vi "PCO_Camera_Type.vi"() -> (0 "PCO_CameraType":T1 {"wCamType" format="%x"; "wCamSubType" format="%x"; "InterfaceType" format="%x"}, 1 "PCO_CameraType_Raw":T2, 2 "Length":u16, 3 "Raw_Length":u16)   [LabVIEW 2019, in "SDK.lvlib" / "Structures.lvlib"]
doc: "Use this template to build a VI to use as a subVI."
uses:
  Structures.lvlib
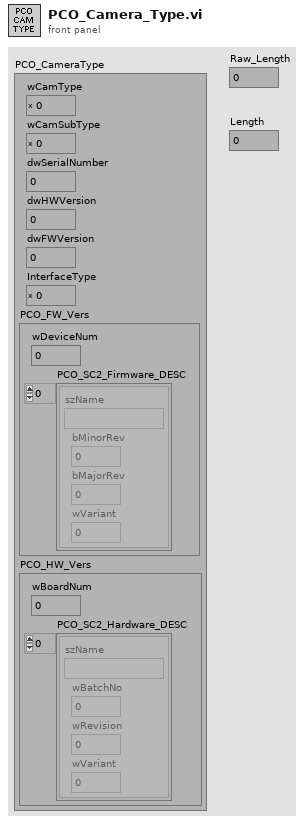
[diagram p1: front panel]
types:
  T1 = cluster{"wCamType":u16, "wCamSubType":u16, "dwSerialNumber":u32, "dwHWVersion":u32, "dwFWVersion":u32, "InterfaceType":u16, "PCO_FW_Vers":cluster{"wDeviceNum":u16, "PCO_SC2_Firmware_DESC":cluster{"szName":string, "bMinorRev":u8, "bMajorRev":u8, "wVariant":u16}[]}, "PCO_HW_Vers":cluster{"wBoardNum":u16, "PCO_SC2_Hardware_DESC":cluster{"szName":string, "wBatchNo":u16, "wRevision":u16, "wVariant":u16}[]}}
  T2 = cluster{"wSize":u16, "wCamType":u16, "wCamSubType":u16, "zzwAlignDummy1":u16, "dwSerialNumber":u32, "dwHWVersion":u32, "dwFWVersion":u32, "wInterfaceType":u16, "PCO_FW_Vers_Raw":cluster{"wDeviceNum":u16, "PCO_SC2_Firmware_DESC":cluster{"PCO_SC2_FW_Desc_Raw":cluster{"szName":cluster{u8, u8, u8, u8, u8, u8, u8, u8, u8, u8, u8, u8, u8, u8, u8, u8}, "bMinorRev":u8, "bMajorRev":u8, "wVariant":u16, "zzwDummy":cluster{u16, u16, u16, u16, u16, u16, u16, u16, u16, u16, u16, u16, u16, u16, u16, u16, u16, u16, u16, u16, u16, u16}}, "PCO_SC2_FW_Desc_Raw":cluster{"szName":cluster{u8, u8, u8, u8, u8, u8, u8, u8, u8, u8, u8, u8, u8, u8, u8, u8}, "bMinorRev":u8, "bMajorRev":u8, "wVariant":u16, "zzwDummy":cluster{u16, u16, u16, u16, u16, u16, u16, u16, u16, u16, u16, u16, u16, u16, u16, u16, u16, u16, u16, u16, u16, u16}}, "PCO_SC2_FW_Desc_Raw":cluster{"szName":cluster{u8, u8, u8, u8, u8, u8, u8, u8, u8, u8, u8, u8, u8, u8, u8, u8}, "bMinorRev":u8, "bMajorRev":u8, "wVariant":u16, "zzwDummy":cluster{u16, u16, u16, u16, u16, u16, u16, u16, u16, u16, u16, u16, u16, u16, u16, u16, u16, u16, u16, u16, u16, u16}}, "PCO_SC2_FW_Desc_Raw":cluster{"szName":cluster{u8, u8, u8, u8, u8, u8, u8, u8, u8, u8, u8, u8, u8, u8, u8, u8}, "bMinorRev":u8, "bMajorRev":u8, "wVariant":u16, "zzwDummy":cluster{u16, u16, u16, u16, u16, u16, u16, u16, u16, u16, u16, u16, u16, u16, u16, u16, u16, u16, u16, u16, u16, u16}}, "PCO_SC2_FW_Desc_Raw":cluster{"szName":cluster{u8, u8, u8, u8, u8, u8, u8, u8, u8, u8, u8, u8, u8, u8, u8, u8}, "bMinorRev":u8, "bMajorRev":u8, "wVariant":u16, "zzwDummy":cluster{u16, u16, u16, u16, u16, u16, u16, u16, u16, u16, u16, u16, u16, u16, u16, u16, u16, u16, u16, u16, u16, u16}}, "PCO_SC2_FW_Desc_Raw":cluster{"szName":cluster{u8, u8, u8, u8, u8, u8, u8, u8, u8, u8, u8, u8, u8, u8, u8, u8}, "bMinorRev":u8, "bMajorRev":u8, "wVariant":u16, "zzwDummy":cluster{u16, u16, u16, u16, u16, u16, u16, u16, u16, u16, u16, u16, u16, u16, u16, u16, u16, u16, u16, u16, u16, u16}}, "PCO_SC2_FW_Desc_Raw":cluster{"szName":cluster{u8, u8, u8, u8, u8, u8, u8, u8, u8, u8, u8, u8, u8, u8, u8, u8}, "bMinorRev":u8, "bMajorRev":u8, "wVariant":u16, "zzwDummy":cluster{u16, u16, u16, u16, u16, u16, u16, u16, u16, u16, u16, u16, u16, u16, u16, u16, u16, u16, u16, u16, u16, u16}}, "PCO_SC2_FW_Desc_Raw":cluster{"szName":cluster{u8, u8, u8, u8, u8, u8, u8, u8, u8, u8, u8, u8, u8, u8, u8, u8}, "bMinorRev":u8, "bMajorRev":u8, "wVariant":u16, "zzwDummy":cluster{u16, u16, u16, u16, u16, u16, u16, u16, u16, u16, u16, u16, u16, u16, u16, u16, u16, u16, u16, u16, u16, u16}}, "PCO_SC2_FW_Desc_Raw":cluster{"szName":cluster{u8, u8, u8, u8, u8, u8, u8, u8, u8, u8, u8, u8, u8, u8, u8, u8}, "bMinorRev":u8, "bMajorRev":u8, "wVariant":u16, "zzwDummy":cluster{u16, u16, u16, u16, u16, u16, u16, u16, u16, u16, u16, u16, u16, u16, u16, u16, u16, u16, u16, u16, u16, u16}}, "PCO_SC2_FW_Desc_Raw":cluster{"szName":cluster{u8, u8, u8, u8, u8, u8, u8, u8, u8, u8, u8, u8, u8, u8, u8, u8}, "bMinorRev":u8, "bMajorRev":u8, "wVariant":u16, "zzwDummy":cluster{u16, u16, u16, u16, u16, u16, u16, u16, u16, u16, u16, u16, u16, u16, u16, u16, u16, u16, u16, u16, u16, u16}}}}, "PCO_HW_Vers_Raw":cluster{"wBoardNum":u16, "PCO_SC2_Hardware_DESC":cluster{"PCO_SC2_HW_Desc_Raw":cluster{"szName":cluster{u8, u8, u8, u8, u8, u8, u8, u8, u8, u8, u8, u8, u8, u8, u8, u8}, "wBatchNo":u16, "wRevision":u16, "wVariant":u16, "zzwDummy":cluster{u16, u16, u16, u16, u16, u16, u16, u16, u16, u16, u16, u16, u16, u16, u16, u16, u16, u16, u16, u16}}, "PCO_SC2_HW_Desc_Raw":cluster{"szName":cluster{u8, u8, u8, u8, u8, u8, u8, u8, u8, u8, u8, u8, u8, u8, u8, u8}, "wBatchNo":u16, "wRevision":u16, "wVariant":u16, "zzwDummy":cluster{u16, u16, u16, u16, u16, u16, u16, u16, u16, u16, u16, u16, u16, u16, u16, u16, u16, u16, u16, u16}}, "PCO_SC2_HW_Desc_Raw":cluster{"szName":cluster{u8, u8, u8, u8, u8, u8, u8, u8, u8, u8, u8, u8, u8, u8, u8, u8}, "wBatchNo":u16, "wRevision":u16, "wVariant":u16, "zzwDummy":cluster{u16, u16, u16, u16, u16, u16, u16, u16, u16, u16, u16, u16, u16, u16, u16, u16, u16, u16, u16, u16}}, "PCO_SC2_HW_Desc_Raw":cluster{"szName":cluster{u8, u8, u8, u8, u8, u8, u8, u8, u8, u8, u8, u8, u8, u8, u8, u8}, "wBatchNo":u16, "wRevision":u16, "wVariant":u16, "zzwDummy":cluster{u16, u16, u16, u16, u16, u16, u16, u16, u16, u16, u16, u16, u16, u16, u16, u16, u16, u16, u16, u16}}, "PCO_SC2_HW_Desc_Raw":cluster{"szName":cluster{u8, u8, u8, u8, u8, u8, u8, u8, u8, u8, u8, u8, u8, u8, u8, u8}, "wBatchNo":u16, "wRevision":u16, "wVariant":u16, "zzwDummy":cluster{u16, u16, u16, u16, u16, u16, u16, u16, u16, u16, u16, u16, u16, u16, u16, u16, u16, u16, u16, u16}}, "PCO_SC2_HW_Desc_Raw":cluster{"szName":cluster{u8, u8, u8, u8, u8, u8, u8, u8, u8, u8, u8, u8, u8, u8, u8, u8}, "wBatchNo":u16, "wRevision":u16, "wVariant":u16, "zzwDummy":cluster{u16, u16, u16, u16, u16, u16, u16, u16, u16, u16, u16, u16, u16, u16, u16, u16, u16, u16, u16, u16}}, "PCO_SC2_HW_Desc_Raw":cluster{"szName":cluster{u8, u8, u8, u8, u8, u8, u8, u8, u8, u8, u8, u8, u8, u8, u8, u8}, "wBatchNo":u16, "wRevision":u16, "wVariant":u16, "zzwDummy":cluster{u16, u16, u16, u16, u16, u16, u16, u16, u16, u16, u16, u16, u16, u16, u16, u16, u16, u16, u16, u16}}, "PCO_SC2_HW_Desc_Raw":cluster{"szName":cluster{u8, u8, u8, u8, u8, u8, u8, u8, u8, u8, u8, u8, u8, u8, u8, u8}, "wBatchNo":u16, "wRevision":u16, "wVariant":u16, "zzwDummy":cluster{u16, u16, u16, u16, u16, u16, u16, u16, u16, u16, u16, u16, u16, u16, u16, u16, u16, u16, u16, u16}}, "PCO_SC2_HW_Desc_Raw":cluster{"szName":cluster{u8, u8, u8, u8, u8, u8, u8, u8, u8, u8, u8, u8, u8, u8, u8, u8}, "wBatchNo":u16, "wRevision":u16, "wVariant":u16, "zzwDummy":cluster{u16, u16, u16, u16, u16, u16, u16, u16, u16, u16, u16, u16, u16, u16, u16, u16, u16, u16, u16, u16}}, "PCO_SC2_HW_Desc_Raw":cluster{"szName":cluster{u8, u8, u8, u8, u8, u8, u8, u8, u8, u8, u8, u8, u8, u8, u8, u8}, "wBatchNo":u16, "wRevision":u16, "wVariant":u16, "zzwDummy":cluster{u16, u16, u16, u16, u16, u16, u16, u16, u16, u16, u16, u16, u16, u16, u16, u16, u16, u16, u16, u16}}}}, "zzWDummy":cluster{u16, u16, u16, u16, u16, u16, u16, u16, u16, u16, u16, u16, u16, u16, u16, u16, u16, u16, u16, u16, u16, u16, u16, u16, u16, u16, u16, u16, u16, u16, u16, u16, u16, u16, u16, u16, u16, u16, u16}}
  T3 = cluster{u16, u16, u16, u16, u16, u16, u16, u16, u16, u16, u16, u16, u16, u16, u16, u16, u16, u16, u16, u16, u16, u16, u16, u16, u16, u16, u16, u16, u16, u16, u16, u16, u16, u16, u16, u16, u16, u16, u16}
  T4 = cluster{"wDeviceNum":u16, "PCO_SC2_Firmware_DESC":cluster{"szName":string, "bMinorRev":u8, "bMajorRev":u8, "wVariant":u16}[]}
  T5 = cluster{"wDeviceNum":u16, "PCO_SC2_Firmware_DESC":cluster{"PCO_SC2_FW_Desc_Raw":cluster{"szName":cluster{u8, u8, u8, u8, u8, u8, u8, u8, u8, u8, u8, u8, u8, u8, u8, u8}, "bMinorRev":u8, "bMajorRev":u8, "wVariant":u16, "zzwDummy":cluster{u16, u16, u16, u16, u16, u16, u16, u16, u16, u16, u16, u16, u16, u16, u16, u16, u16, u16, u16, u16, u16, u16}}, "PCO_SC2_FW_Desc_Raw":cluster{"szName":cluster{u8, u8, u8, u8, u8, u8, u8, u8, u8, u8, u8, u8, u8, u8, u8, u8}, "bMinorRev":u8, "bMajorRev":u8, "wVariant":u16, "zzwDummy":cluster{u16, u16, u16, u16, u16, u16, u16, u16, u16, u16, u16, u16, u16, u16, u16, u16, u16, u16, u16, u16, u16, u16}}, "PCO_SC2_FW_Desc_Raw":cluster{"szName":cluster{u8, u8, u8, u8, u8, u8, u8, u8, u8, u8, u8, u8, u8, u8, u8, u8}, "bMinorRev":u8, "bMajorRev":u8, "wVariant":u16, "zzwDummy":cluster{u16, u16, u16, u16, u16, u16, u16, u16, u16, u16, u16, u16, u16, u16, u16, u16, u16, u16, u16, u16, u16, u16}}, "PCO_SC2_FW_Desc_Raw":cluster{"szName":cluster{u8, u8, u8, u8, u8, u8, u8, u8, u8, u8, u8, u8, u8, u8, u8, u8}, "bMinorRev":u8, "bMajorRev":u8, "wVariant":u16, "zzwDummy":cluster{u16, u16, u16, u16, u16, u16, u16, u16, u16, u16, u16, u16, u16, u16, u16, u16, u16, u16, u16, u16, u16, u16}}, "PCO_SC2_FW_Desc_Raw":cluster{"szName":cluster{u8, u8, u8, u8, u8, u8, u8, u8, u8, u8, u8, u8, u8, u8, u8, u8}, "bMinorRev":u8, "bMajorRev":u8, "wVariant":u16, "zzwDummy":cluster{u16, u16, u16, u16, u16, u16, u16, u16, u16, u16, u16, u16, u16, u16, u16, u16, u16, u16, u16, u16, u16, u16}}, "PCO_SC2_FW_Desc_Raw":cluster{"szName":cluster{u8, u8, u8, u8, u8, u8, u8, u8, u8, u8, u8, u8, u8, u8, u8, u8}, "bMinorRev":u8, "bMajorRev":u8, "wVariant":u16, "zzwDummy":cluster{u16, u16, u16, u16, u16, u16, u16, u16, u16, u16, u16, u16, u16, u16, u16, u16, u16, u16, u16, u16, u16, u16}}, "PCO_SC2_FW_Desc_Raw":cluster{"szName":cluster{u8, u8, u8, u8, u8, u8, u8, u8, u8, u8, u8, u8, u8, u8, u8, u8}, "bMinorRev":u8, "bMajorRev":u8, "wVariant":u16, "zzwDummy":cluster{u16, u16, u16, u16, u16, u16, u16, u16, u16, u16, u16, u16, u16, u16, u16, u16, u16, u16, u16, u16, u16, u16}}, "PCO_SC2_FW_Desc_Raw":cluster{"szName":cluster{u8, u8, u8, u8, u8, u8, u8, u8, u8, u8, u8, u8, u8, u8, u8, u8}, "bMinorRev":u8, "bMajorRev":u8, "wVariant":u16, "zzwDummy":cluster{u16, u16, u16, u16, u16, u16, u16, u16, u16, u16, u16, u16, u16, u16, u16, u16, u16, u16, u16, u16, u16, u16}}, "PCO_SC2_FW_Desc_Raw":cluster{"szName":cluster{u8, u8, u8, u8, u8, u8, u8, u8, u8, u8, u8, u8, u8, u8, u8, u8}, "bMinorRev":u8, "bMajorRev":u8, "wVariant":u16, "zzwDummy":cluster{u16, u16, u16, u16, u16, u16, u16, u16, u16, u16, u16, u16, u16, u16, u16, u16, u16, u16, u16, u16, u16, u16}}, "PCO_SC2_FW_Desc_Raw":cluster{"szName":cluster{u8, u8, u8, u8, u8, u8, u8, u8, u8, u8, u8, u8, u8, u8, u8, u8}, "bMinorRev":u8, "bMajorRev":u8, "wVariant":u16, "zzwDummy":cluster{u16, u16, u16, u16, u16, u16, u16, u16, u16, u16, u16, u16, u16, u16, u16, u16, u16, u16, u16, u16, u16, u16}}}}
  T6 = cluster{"wBoardNum":u16, "PCO_SC2_Hardware_DESC":cluster{"szName":string, "wBatchNo":u16, "wRevision":u16, "wVariant":u16}[]}
  T7 = cluster{"wBoardNum":u16, "PCO_SC2_Hardware_DESC":cluster{"PCO_SC2_HW_Desc_Raw":cluster{"szName":cluster{u8, u8, u8, u8, u8, u8, u8, u8, u8, u8, u8, u8, u8, u8, u8, u8}, "wBatchNo":u16, "wRevision":u16, "wVariant":u16, "zzwDummy":cluster{u16, u16, u16, u16, u16, u16, u16, u16, u16, u16, u16, u16, u16, u16, u16, u16, u16, u16, u16, u16}}, "PCO_SC2_HW_Desc_Raw":cluster{"szName":cluster{u8, u8, u8, u8, u8, u8, u8, u8, u8, u8, u8, u8, u8, u8, u8, u8}, "wBatchNo":u16, "wRevision":u16, "wVariant":u16, "zzwDummy":cluster{u16, u16, u16, u16, u16, u16, u16, u16, u16, u16, u16, u16, u16, u16, u16, u16, u16, u16, u16, u16}}, "PCO_SC2_HW_Desc_Raw":cluster{"szName":cluster{u8, u8, u8, u8, u8, u8, u8, u8, u8, u8, u8, u8, u8, u8, u8, u8}, "wBatchNo":u16, "wRevision":u16, "wVariant":u16, "zzwDummy":cluster{u16, u16, u16, u16, u16, u16, u16, u16, u16, u16, u16, u16, u16, u16, u16, u16, u16, u16, u16, u16}}, "PCO_SC2_HW_Desc_Raw":cluster{"szName":cluster{u8, u8, u8, u8, u8, u8, u8, u8, u8, u8, u8, u8, u8, u8, u8, u8}, "wBatchNo":u16, "wRevision":u16, "wVariant":u16, "zzwDummy":cluster{u16, u16, u16, u16, u16, u16, u16, u16, u16, u16, u16, u16, u16, u16, u16, u16, u16, u16, u16, u16}}, "PCO_SC2_HW_Desc_Raw":cluster{"szName":cluster{u8, u8, u8, u8, u8, u8, u8, u8, u8, u8, u8, u8, u8, u8, u8, u8}, "wBatchNo":u16, "wRevision":u16, "wVariant":u16, "zzwDummy":cluster{u16, u16, u16, u16, u16, u16, u16, u16, u16, u16, u16, u16, u16, u16, u16, u16, u16, u16, u16, u16}}, "PCO_SC2_HW_Desc_Raw":cluster{"szName":cluster{u8, u8, u8, u8, u8, u8, u8, u8, u8, u8, u8, u8, u8, u8, u8, u8}, "wBatchNo":u16, "wRevision":u16, "wVariant":u16, "zzwDummy":cluster{u16, u16, u16, u16, u16, u16, u16, u16, u16, u16, u16, u16, u16, u16, u16, u16, u16, u16, u16, u16}}, "PCO_SC2_HW_Desc_Raw":cluster{"szName":cluster{u8, u8, u8, u8, u8, u8, u8, u8, u8, u8, u8, u8, u8, u8, u8, u8}, "wBatchNo":u16, "wRevision":u16, "wVariant":u16, "zzwDummy":cluster{u16, u16, u16, u16, u16, u16, u16, u16, u16, u16, u16, u16, u16, u16, u16, u16, u16, u16, u16, u16}}, "PCO_SC2_HW_Desc_Raw":cluster{"szName":cluster{u8, u8, u8, u8, u8, u8, u8, u8, u8, u8, u8, u8, u8, u8, u8, u8}, "wBatchNo":u16, "wRevision":u16, "wVariant":u16, "zzwDummy":cluster{u16, u16, u16, u16, u16, u16, u16, u16, u16, u16, u16, u16, u16, u16, u16, u16, u16, u16, u16, u16}}, "PCO_SC2_HW_Desc_Raw":cluster{"szName":cluster{u8, u8, u8, u8, u8, u8, u8, u8, u8, u8, u8, u8, u8, u8, u8, u8}, "wBatchNo":u16, "wRevision":u16, "wVariant":u16, "zzwDummy":cluster{u16, u16, u16, u16, u16, u16, u16, u16, u16, u16, u16, u16, u16, u16, u16, u16, u16, u16, u16, u16}}, "PCO_SC2_HW_Desc_Raw":cluster{"szName":cluster{u8, u8, u8, u8, u8, u8, u8, u8, u8, u8, u8, u8, u8, u8, u8, u8}, "wBatchNo":u16, "wRevision":u16, "wVariant":u16, "zzwDummy":cluster{u16, u16, u16, u16, u16, u16, u16, u16, u16, u16, u16, u16, u16, u16, u16, u16, u16, u16, u16, u16}}}}
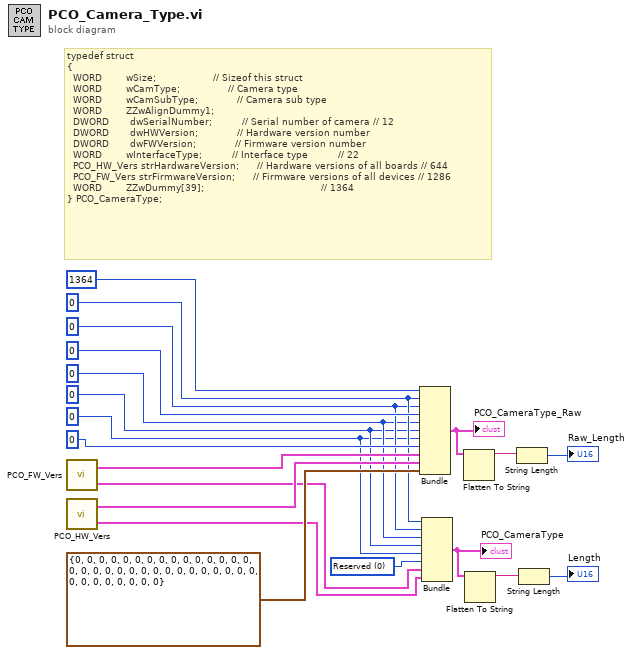
[diagram p0: block diagram]
diagram:
  w9 = u16 0 items=["Reserved", "Firewire/IEEE 1394", "CameraLink", "USB", "Ethernet", "Serial interface", "USB3", "CameraLink HS", "Coaxpress", "USB3.1 Gen1", "Reserved"] ("InterfaceType")
  w10 = u32 0 ("dwFWVersion")
  w11 = u32 0 ("dwHWVersion")
  w12 = u32 0 ("dwSerialNumber")
  w13 = u16 0 ("wCamSubType")
  w14 = u16 0 ("wCamType")
  # "typedef struct\n{\n  WORD        wSize;                   // Sizeof this struct\n  WORD        wCamType;                // Camera type\n  WORD        wCamSubType;             // Camera sub type\n  WORD        ZZwAlignDummy1;\n  DWORD       dwSerialNumber;          // Serial number of camera // 12\n  DWORD       dwHWVersion;             // Hardware version number\n  DWORD       dwFWVersion;             // Firmware version number\n  WORD        wInterfaceType;          // Interface type          // 22\n  PCO_HW_Vers strHardwareVersion;      // Hardware versions of all boards // 644\n  PCO_FW_Vers strFirmwareVersion;      // Firmware versions of all devices // 1286\n  WORD        ZZwDummy[39];                                       // 1364\n} PCO_CameraType;"
  n1 = call "PCO_FW_Vers.vi"() -> ("PCO_FW_Vers"=w8:T4, "PCO_FW_Vers_Raw"=w18:T5)  [unwired: 4 in, 2 out]
  n2 = call "PCO_HW_Vers.vi"() -> ("PCO_HW_Vers"=w7:T6, "PCO_HW_Vers_Raw"=w19:T7)  [unwired: 4 in, 2 out]
  n3 = Bundle("wSize"=u16 1364, "wCamType"=w14, "wCamSubType"=w13, "zzwAlignDummy1"=u16 0, "dwSerialNumber"=w12, "dwHWVersion"=w11, "dwFWVersion"=w10, "wInterfaceType"=u16 0, "PCO_FW_Vers_Raw"=w18, "PCO_HW_Vers_Raw"=w19, "zzWDummy"=T3 {0, 0, 0, 0, 0, 0, 0, 0, 0, 0, 0, 0, 0, 0, 0, 0, 0, 0, 0, 0, 0, 0, 0, 0, 0, 0, 0, 0, 0, 0, 0, 0, 0, 0, 0, 0, 0, 0, 0}) -> (w1:T2)  [unwired: 1 in]
  "PCO_CameraType_Raw" <- w1
  n4 = Bundle("wCamType"=w14, "wCamSubType"=w13, "dwSerialNumber"=w12, "dwHWVersion"=w11, "dwFWVersion"=w10, "InterfaceType"=w9, "PCO_FW_Vers"=w8, "PCO_HW_Vers"=w7) -> (w6:T1)  [unwired: 1 in]
  "PCO_CameraType" <- w6
  n5 = Flatten To String(anything=w1) -> (data string=w4:string)  [unwired: 3 in, 2 out]
  n6 = Flatten To String(anything=w6) -> (data string=w5:string)  [unwired: 3 in, 2 out]
  n7 = String Length(string=w4) -> (length=→"Raw_Length":i32)
  n8 = String Length(string=w5) -> (length=→"Length":i32)
